vi "Server_LabView.vi"() -> ()   [LabVIEW 2021]
panel:
  out "number (0 to 1)":dbl
  in  "Event":string
  out "Array":dbl[][](array[numeric])
  out "data string":string
  out "Array of element extracted\nfrom the array depending on \nthe coordinates given":dbl[](array[numeric])
  out "length":string
  out "Iteration":i32
  out "Command\nreceived":string
  out "error out":errorcluster
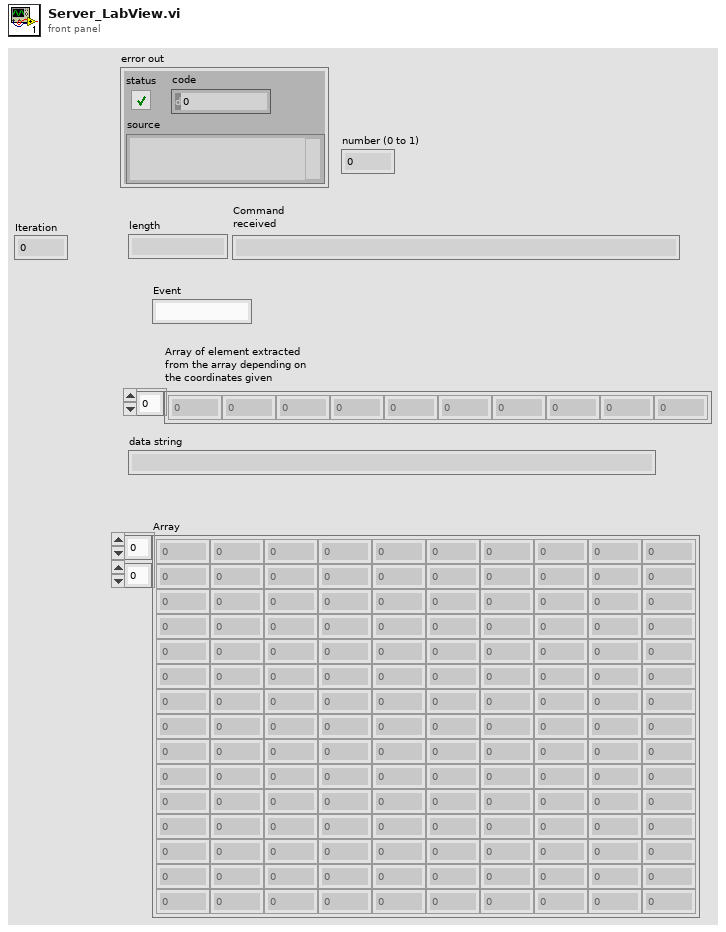
[diagram p1: front panel]
types:
  T1 = enum16{"big-endian, network order", "native, host order", "little-endian"}
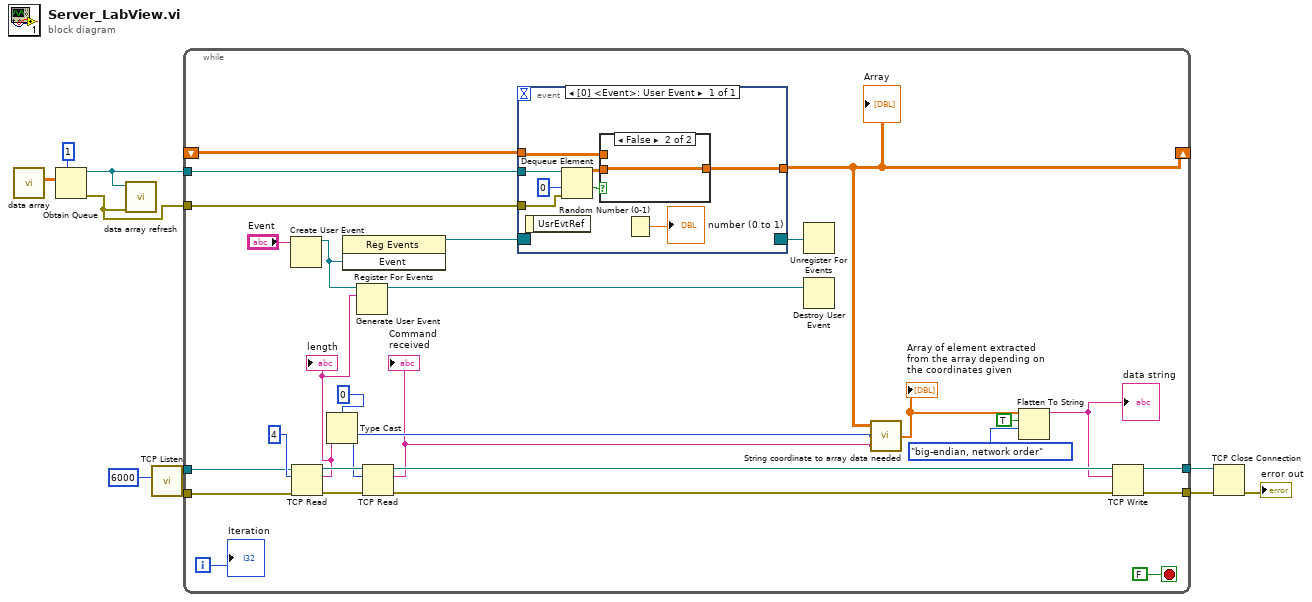
[diagram p0: block diagram]
diagram:
  n1 = call "data array.vi"() -> ("Array"=w10:dbl[][])  [unwired: 11 in]
  n2 = Obtain Queue(max queue size (-1, unlimited)=1, element data type=w10) -> (queue out=w2:refnum<queue>, error out=w1:errorcluster)  [unwired: 3 in, 1 out]
  n3 = call "data array refresh.vi"("error in (no error)"=w1, "queue out"=w2) -> ()  [unwired: 10 in]
  n4 = call <vilib>:"TCP Listen.vi"("port"=u16 6000) -> ("error out"=w4:errorcluster, "connection ID"=w3:refnum<k5>)  [unwired: 6 in, 3 out]
  n5 = while {
    tunnel: w2 -> [w17]
    tunnel: w1 -> [w16]
    tunnel: [w32] -> w7
    tunnel: [w31] -> w6
    tunnel: w4 -> [w30]
    tunnel: w3 -> [w29]
    shift-right: [w14] -> _
    shift-left: _ -> [w18]
    i -> [w34]
    stop <- FALSE stop-if-true
    n6 = Create User Event(user event datatype="Event") -> (user event=w21:refnum<user-event>)  [unwired: 1 in, 1 out]
    n7 = TCP Read(connection ID=w29, bytes to read=4, error in (no error)=w30) -> (connection ID out=w38:refnum<k5>, data out=w15:string, error out=w37:errorcluster)  [unwired: 2 in]
    "length" <- w15
    n8 = Type Cast(type=0, x=w15) -> (*(type *) &x=w13:i32)
    n9 = register-events(w21) -> (reference out=w22:refnum<event-registration>)  [unwired: 2 in, 1 out]
    n10 = Generate User Event(user event=w21, event data cluster=w15) -> (user event out=w19:refnum<user-event>)  [unwired: 2 in, 1 out]
    n11 = TCP Read(connection ID=w38, bytes to read=w13, error in (no error)=w37) -> (connection ID out=w28:refnum<k5>, data out=w12:string, error out=w27:errorcluster)  [unwired: 2 in]
    "Command\nreceived" <- w12
    n12 = event shown="[0] <Event>: User Event" {
      selector: w22 -> [_]
      dyn-events: [_] -> w20
      timeout: _ -> [_]
      tunnel: w18 -> [w44]
      tunnel: w17 -> [w43]
      tunnel: w16 -> [w41]
      tunnel: [w40] -> w14
      event User Event {
        n13 = event-data() -> ()  [unwired: 1 in, 1 out]
        n14 = Dequeue Element(queue=w43, timeout in ms (-1)=0, error in (no error)=w41) -> (element=w46:dbl[][], timed out?=w45:bool)  [unwired: 2 out]
        n15 = case shown="False" w45 {
          tunnel: w46 -> [_ w48]
          tunnel: w44 -> [w47 _]
          tunnel: [w47 w48] -> w40
          frame True {
          }
          frame False {
          }
        }
        n16 = Random Number (0-1)() -> (number: 0 to 1=→"number (0 to 1)":dbl)
      }
    }
    "Array" <- w14
    n17 = Unregister For Events(event registration refnum=w20) -> ()  [unwired: 1 in, 1 out]
    n18 = Destroy User Event(user event=w19) -> ()  [unwired: 1 in, 1 out]
    n19 = call "String coordinate to array data needed.vi"("Input string"=w12, "Number of coordinates to extract"=w13, "Array"=w14) -> ("Array of element extracted\nfrom the data array depending \non the coordinates given"=w11:dbl[])
    "Array of element extracted\nfrom the array depending on \nthe coordinates given" <- w11
    n20 = Flatten To String(anything=w11, prepend array or string size? (T)=TRUE, byte order (0:big-endian, network order)=T1."big-endian, network order") -> (data string=w24:string)  [unwired: 1 in, 2 out]
    "data string" <- w24
    n21 = TCP Write(connection ID=w28, data in=w24, error in (no error)=w27) -> (connection ID out=w31:refnum<k5>, error out=w32:errorcluster)  [unwired: 1 in, 1 out]
    "Iteration" <- w34
  }
  n22 = TCP Close Connection(connection ID=w6, error in (no error)=w7) -> (error out=→"error out":errorcluster)  [unwired: 1 in, 1 out]
